vi "json Parse I32 - string path.vi"(8 "error in (no error)":errorcluster, 9 "default":i32, 10 "path":string, 11 "JSON Document in":refnum<class "JSON Document.lvclass">) -> (0 "error out":errorcluster, 1 "defaulted?":bool, 2 "value":i32, 3 "JSON Document out":refnum<class "JSON Document.lvclass">)   [LabVIEW 2015, in "JSON Document.lvclass"]
uses:
  JSON Document.lvclass
  JSON Document.lvclass/JSON Document.ctl
  json query/json Query - string path.vi
  rapidjson wrapper/rapidjson wrapper.lvlib
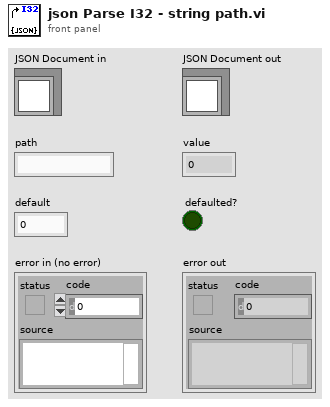
[diagram p1: front panel]
types:
  T1 = typedef "rapidjson wrapper.lvlib/jsonType.ctl" = enum16{"Null", "False", "True", "Object", "Array", "String", "Number"}
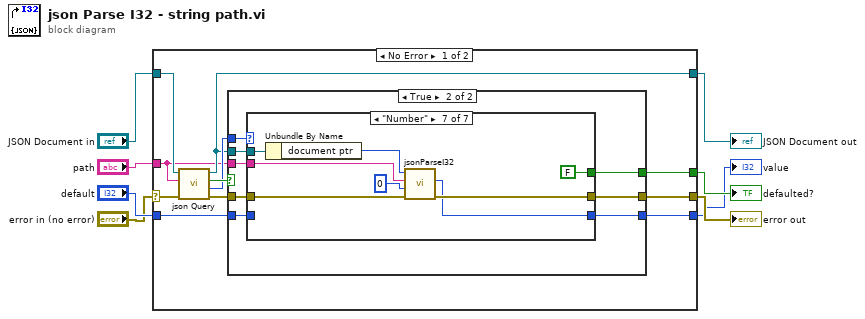
[diagram p0: block diagram]
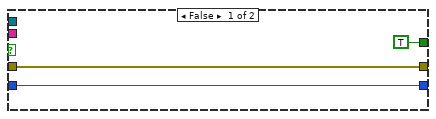
[diagram p2: hidden frame]
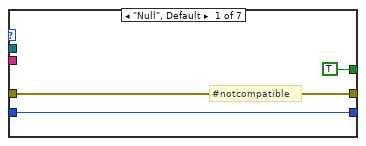
[diagram p3: hidden frame]
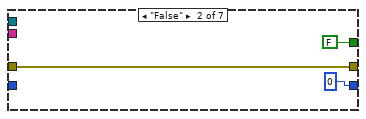
[diagram p4: hidden frame]
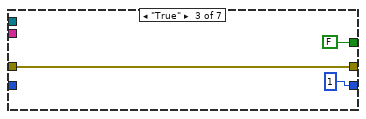
[diagram p5: hidden frame]
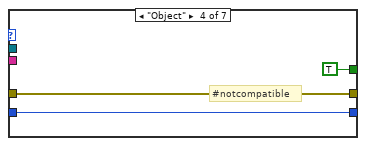
[diagram p6: hidden frame]
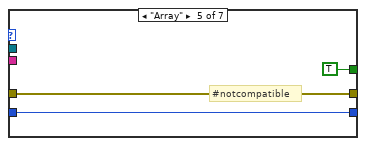
[diagram p7: hidden frame]
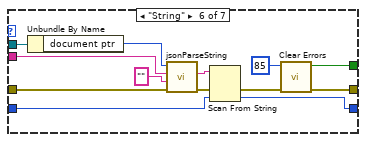
[diagram p8: hidden frame]
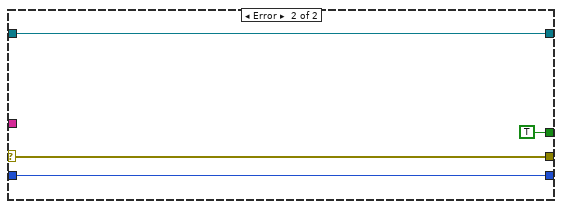
[diagram p9: hidden frame]
diagram:
  n1 = case shown="No Error" "error in (no error)" {
    selector: "error in (no error)" -> [w18 w70]
    tunnel: [w13 w70] -> w6
    tunnel: [w11 w69] -> w8
    tunnel: "JSON Document in" -> [w19 w69]
    tunnel: "default" -> [w15 w68]
    tunnel: "path" -> [w9 _]
    tunnel: [w16 w68] -> w5
    tunnel: [w10 TRUE ("specific error cleared?")] -> w7
    frame No Error {
      n2 = call-poly "json Query.vi"("error in (no error)"=w18, "path"=w9, "JSON Document in"=w19) -> ("error out"=w14:errorcluster, "type"=w12:T1, "found?"=w17:bool, "JSON Document out"=w11:refnum<class "JSON Document.lvclass">)  [unwired: 5 in]
      n3 = case shown="True" w17 {
        tunnel: [w22 w28] -> w16
        tunnel: w15 -> [w22 w29]
        tunnel: w11 -> [_ w27]
        tunnel: w14 -> [w21 w26]
        tunnel: [w21 w25] -> w13
        tunnel: w12 -> [_ w30]
        tunnel: [TRUE ("found?") w24] -> w10
        tunnel: w9 -> [_ w23]
        frame False {
        }
        frame True {
          n4 = case shown="\"Number\"" w30 {
            tunnel: w29 -> [w33 _ _ w42 w45 w52 _]
            tunnel: [w33 0 ("value") 1 ("value") w42 w45 w51 w60] -> w28
            tunnel: w27 -> [_ _ _ _ _ w58 w66]
            tunnel: w26 -> [w32 w36 w39 w41 w44 w57 w65]
            tunnel: [w32 w36 w39 w41 w44 w46 w63] -> w25
            tunnel: [TRUE ("found?") FALSE ("specific error cleared?") FALSE ("default") TRUE ("found?") TRUE ("found?") w47 FALSE ("specific error cleared?")] -> w24
            tunnel: w23 -> [_ _ _ _ _ w54 w62]
            frame "Null", Default {
              # "#notcompatible"
            }
            frame "False" {
            }
            frame "True" {
            }
            frame "Object" {
              # "#notcompatible"
            }
            frame "Array" {
              # "#notcompatible"
            }
            frame "String" {
              n5 = Unbundle By Name(w58) -> ("document ptr"=w56:i64)
              n6 = call "jsonParseString.vi"("error in (no error)"=w57, "default"="", "path"=w54, "d in"=w56) -> ("error out"=w50:errorcluster, "value"=w53:string)  [unwired: 4 in, 2 out]
              n7 = Scan From String(input string=w53, error in=w50, default 1=w52) -> (error out=w49:errorcluster, output 1=w51:i32)  [unwired: 2 in, 2 out]
              n8 = call <vilib>:"Clear Errors.vi"("error in (no error)"=w49, "specific error code to clear (0: all)"=85) -> ("error out"=w46:errorcluster, "specific error cleared?"=w47:bool)  [unwired: 4 in]
            }
            frame "Number" {
              n9 = Unbundle By Name(w66) -> ("document ptr"=w64:i64)
              n10 = call "jsonParseI32.vi"("error in (no error)"=w65, "default"=0, "path"=w62, "d in"=w64) -> ("error out"=w63:errorcluster, "value"=w60:i32)  [unwired: 4 in, 2 out]
            }
          }
        }
      }
    }
    frame Error {
    }
  }
  "error out" <- w6
  "JSON Document out" <- w8
  "value" <- w5
  "defaulted?" <- w7
